vi "Subset Buffers.vi"(6 "engine buffer offset":u64 format="%d bytes", 7 "string buffer offset":u64 format="%d bytes", 8 "error in (no error)":errorcluster, 9 "engine buffer size":u64 format="%d bytes", 10 "string buffer size":u64 format="%d bytes", 11 "Buffers in":refnum<class "Buffers.lvclass">) -> (0 "error out":errorcluster, 2 "subset Buffers":refnum<class "Buffers.lvclass">, 3 "Buffers out":refnum<class "Buffers.lvclass">, 4 "engine buffer offset +size":u64 format="%d bytes", 5 "string buffer offset + size":u64 format="%d bytes")   [LabVIEW 2019, in "DSF Core.lvlib" / "Buffers.lvclass"]
uses:
  Buffers.lvclass
  Buffers.lvclass/Buffers.ctl
  <vilib>/NI/Memory Manager/Classes/Pointer/Pointer.lvclass/Pointer.ctl
  Buffer/Buffer.lvclass/Buffer.ctl
  <vilib>/NI/Memory Manager/Classes/Pointer/Subset.vi
  Buffer/Set Buffer Offset.vi
  <vilib>/NI/Memory Manager/Classes/Pointer/Set Size.vi
  <vilib>/NI/Memory Manager/Classes/Pointer/Get Address.vi
  <vilib>/NI/Memory Manager/Classes/Pointer/Encapsulate.vi
  <vilib>/NI/Memory Manager/Classes/Pointer/Check Null Pointer.vi
  <vilib>/NI/Memory Manager/Classes/Pointer/Check Length.vi
  <vilib>/NI/Memory Manager/Classes/Pointer/Set Address.vi
  <vilib>/NI/Memory Manager/Classes/Pointer/Set Internal.vi
  <vilib>/NI/Memory Manager/Classes/Pointer/Errors.vi
  <vilib>/NI/Memory Manager/Classes/Pointer/Null Pointer.vi
  <vilib>/NI/Memory Manager/Classes/Pointer/Is Null.vi
  <vilib>/NI/Memory Manager/Classes/Pointer/Get Size.vi
  <vilib>/NI/Memory Manager/Classes/Pointer/Check Bounds (Pointer).vi
  <vilib>/NI/Memory Manager/Classes/Pointer/Create Error.vi
  <vilib>/NI/Memory Manager/Classes/Pointer/Out of Bounds.vi
  <vilib>/NI/Memory Manager/VIs/New Error Cluster.vi
  <vilib>/NI/Memory Manager/VIs/New Error Cluster (512B).vi
  <vilib>/NI/Memory Manager/VIs/Set Error Status.vi
  <vilib>/NI/Memory Manager/VIs/Set Error Code.vi
  <vilib>/NI/Memory Manager/VIs/Set Error Source.vi
  <vilib>/NI/Memory Manager/Constants/Constants.vi
  <vilib>/NI/Memory Manager/Constants/Library Name.vi
  <vilib>/NI/Memory Manager/Classes/Pointer/Pointer Error Info.vi
  <vilib>/NI/Memory Manager/VIs/Write String to Source.vi
  <vilib>/NI/Memory Manager/Constants/Pointer Class Name.vi
  <vilib>/NI/Memory Manager/Classes/Pointer/Write Pointer Size to Error.vi
  <vilib>/NI/Memory Manager/VIs/Write Numeric to Source.vi
  <vilib>/NI/Memory Manager/VIs/Write Numeric Scalar to Source (Base10 U64).vi
  Buffer/Buffer.lvclass
  C:/Program Files (x86)/National Instruments/LabVIEW 2019/vi.lib/NI/Memory Manager/Classes/Pointer/Pointer.lvclass
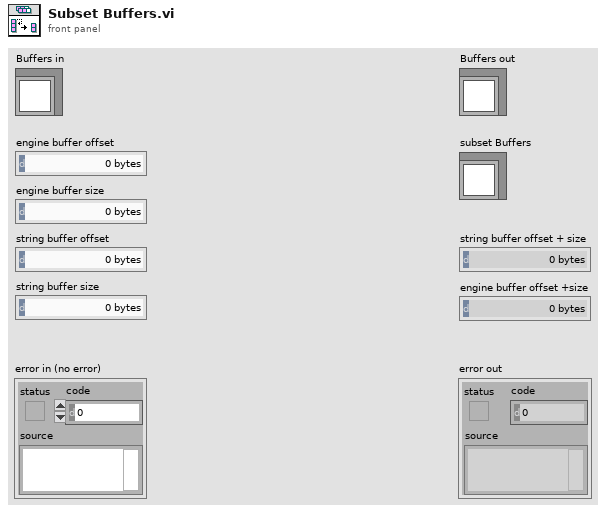
[diagram p1: front panel]
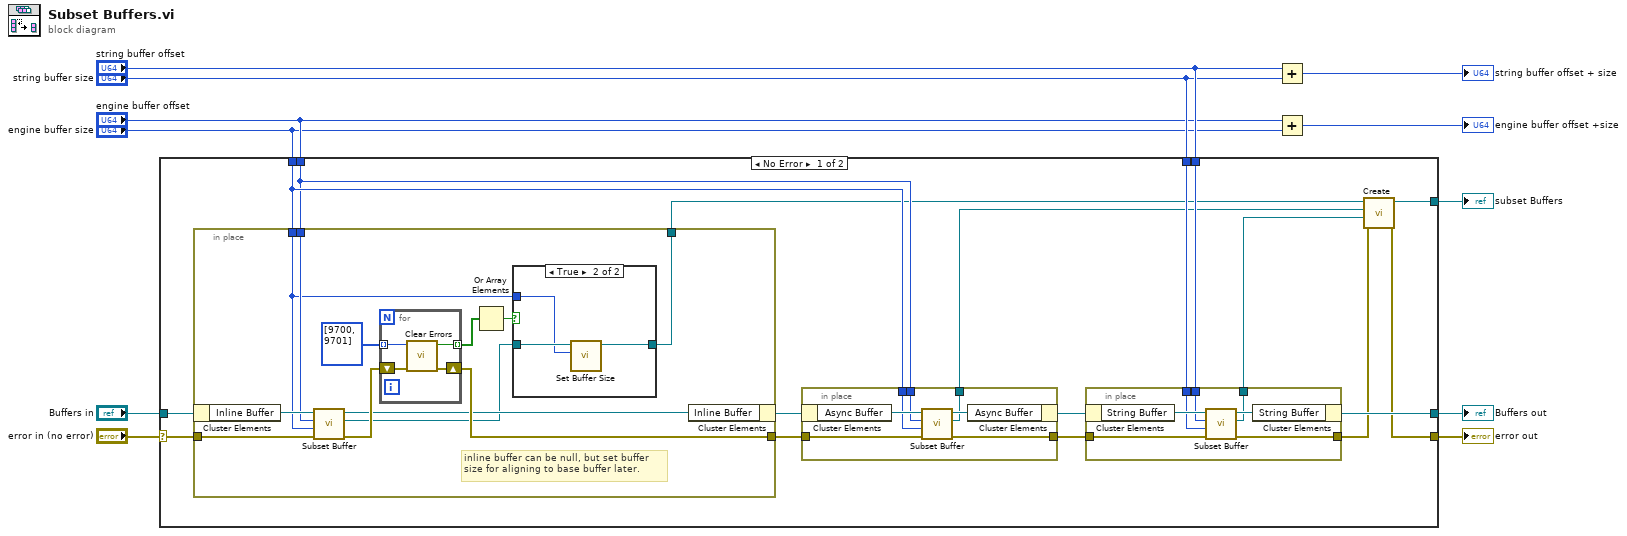
[diagram p0: block diagram]
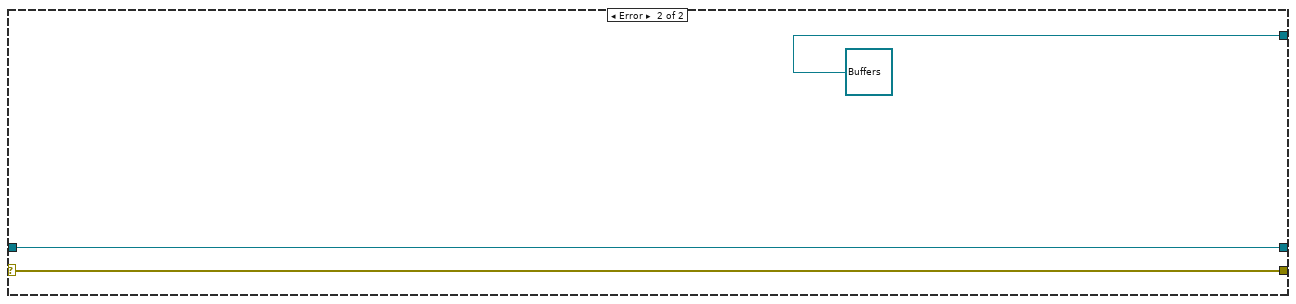
[diagram p3: hidden frame]
diagram:
  n1 = case shown="No Error" "error in (no error)" {
    selector: "error in (no error)" -> [w17 w65]
    tunnel: [w28 refnum<class "Buffers.lvclass"> refnum ("Buffers out")] -> w11
    tunnel: "Buffers in" -> [w27 w64]
    tunnel: [w26 w64] -> w9
    tunnel: "string buffer offset" -> [w25 _]
    tunnel: "string buffer size" -> [w24 _]
    tunnel: "engine buffer offset" -> [w13 _]
    tunnel: "engine buffer size" -> [w14 _]
    tunnel: [w23 w65] -> w2
    frame No Error {
      n2 = in-place {
        in-place-border: w17 -> [w38]
        in-place-border: w13 -> [w37]
        in-place-border: w14 -> [w33]
        in-place-border: [w40] -> w16
        in-place-border: [w30] -> w12
        # "inline buffer can be null, but set buffer size for aligning to base buffer later."
        n3 = in-place-cluster #1(w27) -> ("Inline Buffer"=w39:refnum<class "Buffer.lvclass">)
        n4 = call "Subset Buffer.vi"("error in (no error)"=w38, "size"=w33, "offset"=w37, "Buffer in"=w39) -> ("error out"=w35:errorcluster, "subset Buffer"=w31:refnum<class "Buffer.lvclass">, "Buffer out"=w32:refnum<class "Buffer.lvclass">)  [unwired: 4 in, 1 out]
        n5 = for {
          tunnel: i32[] [9700, 9701] ("specific error code to clear (0: all)") -> [w46] mode=indexing
          shift-right: [w48] -> w40
          shift-left: w35 -> [w47]
          tunnel: [w45] -> w29 mode=indexing
          n6 = call <vilib>:"Clear Errors.vi"("error in (no error)"=w47, "specific error code to clear (0: all)"=w46) -> ("error out"=w48:errorcluster, "specific error cleared?"=w45:bool)  [unwired: 4 in]
        }
        n7 = Or Array Elements(Boolean array=w29) -> (logical OR=w34:bool)
        n8 = case shown="True" w34 {
          tunnel: w31 -> [w41 w44]
          tunnel: [w41 w43] -> w30
          tunnel: w33 -> [_ w42]
          frame False {
          }
          frame True {
            n9 = call "Set Buffer Size.vi"("buffer size"=w42, "Buffer in"=w44) -> ("Buffer out"=w43:refnum<class "Buffer.lvclass">)  [unwired: 9 in]
          }
        }
        n10 = in-place-cluster #1("Inline Buffer"=w32) -> (w15:refnum<class "Buffers.lvclass">)
      }
      n11 = in-place {
        in-place-border: w16 -> [w60]
        in-place-border: [w59] -> w21
        in-place-border: w13 -> [w58]
        in-place-border: w14 -> [w57]
        in-place-border: [w56] -> w18
        n12 = in-place-cluster #2(w15) -> ("Async Buffer"=w62:refnum<class "Buffer.lvclass">)
        n13 = call "Subset Buffer.vi"("error in (no error)"=w60, "size"=w57, "offset"=w58, "Buffer in"=w62) -> ("error out"=w59:errorcluster, "subset Buffer"=w56:refnum<class "Buffer.lvclass">, "Buffer out"=w61:refnum<class "Buffer.lvclass">)  [unwired: 4 in, 1 out]
        n14 = in-place-cluster #2("Async Buffer"=w61) -> (w22:refnum<class "Buffers.lvclass">)
      }
      n15 = in-place {
        in-place-border: w21 -> [w53]
        in-place-border: [w52] -> w20
        in-place-border: w25 -> [w50]
        in-place-border: w24 -> [w51]
        in-place-border: [w49] -> w19
        n16 = in-place-cluster #3(w22) -> ("String Buffer"=w55:refnum<class "Buffer.lvclass">)
        n17 = call "Subset Buffer.vi"("error in (no error)"=w53, "size"=w51, "offset"=w50, "Buffer in"=w55) -> ("error out"=w52:errorcluster, "subset Buffer"=w49:refnum<class "Buffer.lvclass">, "Buffer out"=w54:refnum<class "Buffer.lvclass">)  [unwired: 4 in, 1 out]
        n18 = in-place-cluster #3("String Buffer"=w54) -> (w26:refnum<class "Buffers.lvclass">)
      }
      n19 = call "Create.vi"("error in (no error)"=w20, "String Buffer (null)"=w19, "Async Buffer (null)"=w18, "Inline Buffer (null)"=w12) -> ("error out"=w23:errorcluster, "Buffers out"=w28:refnum<class "Buffers.lvclass">)  [unwired: 6 in]
    }
    frame Error {
    }
  }
  "error out" <- w2
  "Buffers out" <- w9
  "subset Buffers" <- w11
  n20 = Add(x="string buffer offset", y="string buffer size") -> (x+y=→"string buffer offset + size":u64)
  n21 = Add(x="engine buffer offset", y="engine buffer size") -> (x+y=→"engine buffer offset +size":u64)
